vi "Position FG.vi"(4 "Parameter":T1(ring), 5 "Get / Set (T=Set)":bool, 6 "Level":dbl, 7 "Channel In":u32, 8 "Slope":bool, 9 "Source":bool, 10 "Volts / Div In":u32, 11 "Time Base In":u32) -> (3 "Parameters":T2)   [LabVIEW 2009]
panel:
  # "Oscilloscope Functional Global Variable"
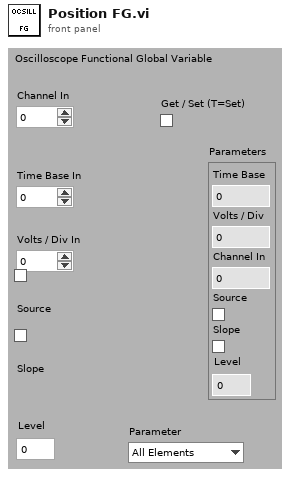
[diagram p1: front panel]
types:
  T1 = enum16{"All Elements", "Channel", "Source", "Level", "Slope", "Time Base", "Volts / Div"}
  T2 = cluster{"Time Base":u32, "Volts / Div":u32, "Channel In":u32, "Source":bool, "Slope":bool, "Level":dbl}
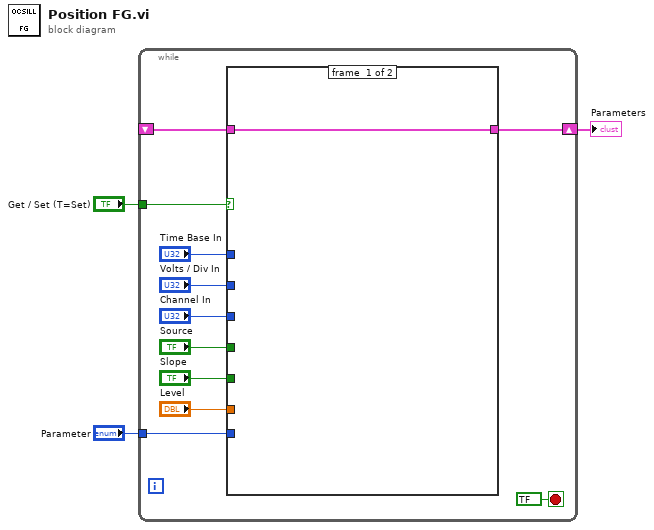
[diagram p0: block diagram]
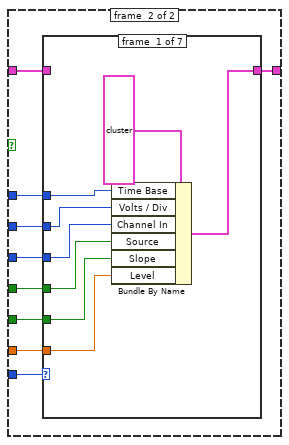
[diagram p2: hidden frame]
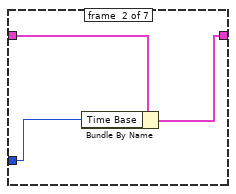
[diagram p3: hidden frame]
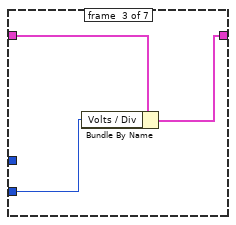
[diagram p4: hidden frame]
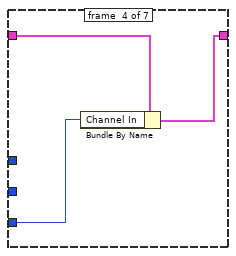
[diagram p5: hidden frame]
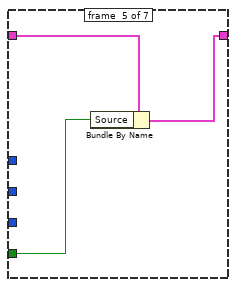
[diagram p6: hidden frame]
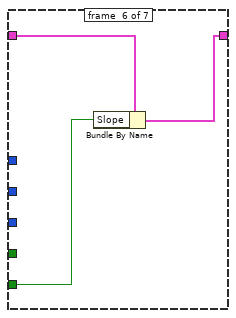
[diagram p7: hidden frame]
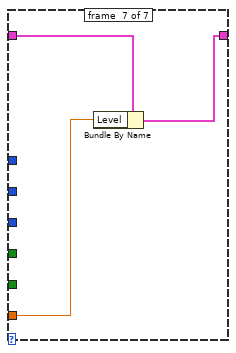
[diagram p8: hidden frame]
diagram:
  n1 = while {
    shift-right: [w12] -> w2
    shift-left: _ -> [w11]
    tunnel: "Get / Set (T=Set)" -> [w13]
    tunnel: "Parameter" -> [w4]
    stop <- bool ? stop-if-true
    n2 = case shown="True" w13 {
      tunnel: [w15 w16] -> w12
      tunnel: w11 -> [w15 w17]
      tunnel: "Time Base In" -> [_ w23]
      tunnel: "Volts / Div In" -> [_ w22]
      tunnel: "Channel In" -> [_ w21]
      tunnel: "Source" -> [_ w20]
      tunnel: "Slope" -> [_ w19]
      tunnel: "Level" -> [_ w18]
      tunnel: w4 -> [_ w24]
      frame #0 {
      }
      frame #1 {
        n3 = case shown="\"Level\"" w24 {
          tunnel: w23 -> [w32 w33 _ _ _ _ _]
          tunnel: w22 -> [w31 _ w36 _ _ _ _]
          tunnel: w21 -> [w29 _ _ w39 _ _ _]
          tunnel: w20 -> [w28 _ _ _ w42 _ _]
          tunnel: w19 -> [w27 _ _ _ _ w45 _]
          tunnel: w18 -> [w26 _ _ _ _ _ w48]
          tunnel: w17 -> [_ w35 w38 w41 w44 w47 w50]
          tunnel: [w25 w34 w37 w40 w43 w46 w49] -> w16
          frame #0 {
            n4 = Bundle By Name(cluster=T2 ? ("Parameters"), "Time Base"=w32, "Volts / Div"=w31, "Channel In"=w29, "Source"=w28, "Slope"=w27, "Level"=w26) -> (w25:T2)
          }
          frame #1 {
            n5 = Bundle By Name(cluster=w35, "Time Base"=w33) -> (w34:T2)
          }
          frame #2 {
            n6 = Bundle By Name(cluster=w38, "Volts / Div"=w36) -> (w37:T2)
          }
          frame #3 {
            n7 = Bundle By Name(cluster=w41, "Channel In"=w39) -> (w40:T2)
          }
          frame #4 {
            n8 = Bundle By Name(cluster=w44, "Source"=w42) -> (w43:T2)
          }
          frame #5 {
            n9 = Bundle By Name(cluster=w47, "Slope"=w45) -> (w46:T2)
          }
          frame #6 {
            n10 = Bundle By Name(cluster=w50, "Level"=w48) -> (w49:T2)
          }
        }
      }
    }
  }
  "Parameters" <- w2
